vi "Prepare Joystick Data for Displays.vi"(11 "Joystick Values":T1) -> (1 "Buttons":T2, 2 "Z Axis":dbl, 3 "Cartesian Data":cluster{"X axis":dbl, "X axis":dbl}[](array[cluster]))   [LabVIEW 2015]
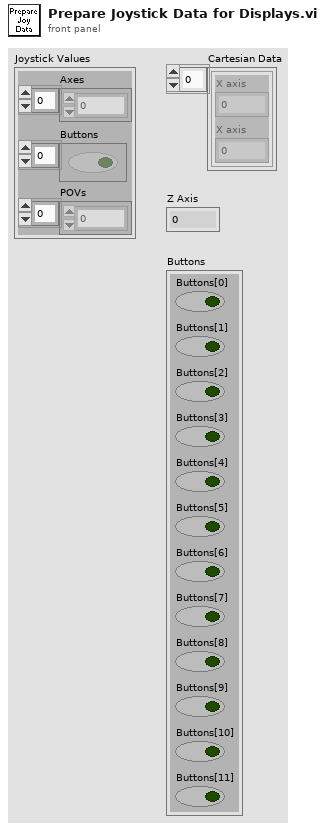
[diagram p1: front panel]
types:
  T1 = cluster{"Axes":dbl[], "Buttons":bool[], "POVs":i16[]}
  T2 = cluster{"Buttons[0]":bool, "Buttons[1]":bool, "Buttons[2]":bool, "Buttons[3]":bool, "Buttons[4]":bool, "Buttons[5]":bool, "Buttons[6]":bool, "Buttons[7]":bool, "Buttons[8]":bool, "Buttons[9]":bool, "Buttons[10]":bool, "Buttons[11]":bool}
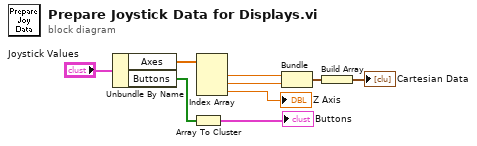
[diagram p0: block diagram]
diagram:
  n1 = Unbundle By Name("Joystick Values") -> ("Axes"=w2:dbl[], "Buttons"=w8:bool[])
  n2 = Array To Cluster(array=w8) -> (cluster=→"Buttons":T2)
  n3 = Index Array(array=w2) -> (element #1=w5:dbl, element #2=w6:dbl, element #3=→"Z Axis":dbl)  [unwired: 3 in]
  n4 = Bundle("X axis"=w5, "X axis"=w6) -> (w4:cluster{"X axis":dbl, "X axis":dbl})  [unwired: 1 in]
  n5 = Build Array(w4) -> (→"Cartesian Data":cluster{"X axis":dbl, "X axis":dbl}[])
